vi "ProdaNG.TestValue.Set.vi"(8 "error in (no error)":errorcluster, 10 "TestValue":T1 {"minimum" format="%#.3f"; "maximum" format="%#.3f"}, 11 "dbHandleIn":i32) -> (0 "error out":errorcluster, 2 "TestValue out":T1 {"minimum" format="%#.3f"; "maximum" format="%#.3f"}, 3 "dbHandle":i32)   [LabVIEW 2016]
doc: "This function returns a product structure for a product, which is identified by a part and a serial number.\nImportant information: The field 'individual' was taken over from the field 'allgemein' of the legacy data directly. Because of this most products have the value 0 further on and only a few the value 1. \nParameter:\nhandle is an Integer, which is returned by the function Login() at the creation of a new connection.\nwabcoPartId is the Id of the part.\nserialNumber is the serial number of the product for the part above.\nproduct is a pointer on a product structure, which is filled if the returncode is 0. The structure must be defined in the calling program.\n\nReturncodes:\n0 No error\n< 0 ORACLE Error code\n6 (ERROR_INVALID_HANDLE) in case of an invalid handle\n1403 Record does not exist"
uses:
  Controls/ProdaNG.TestValue.ctl
  Controls/ProdaNG.TestValueSize.ctl
  prodllNG.dll
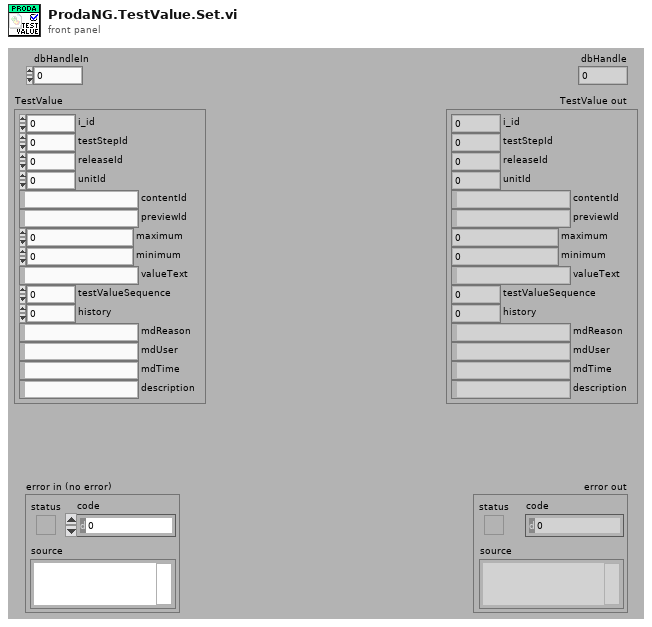
[diagram p1: front panel]
types:
  T1 = typedef "ProdaNG.TestValue.ctl" = cluster{"i_id":i32, "testStepId":i32, "releaseId":i32, "unitId":i32, "contentId":string, "previewId":string, "maximum":dbl, "minimum":dbl, "valueText":string, "testValueSequence":i32, "history":i32, "mdReason":string, "mdUser":string, "mdTime":string, "description":string}
  T2 = typedef "ProdaNG.TestValueSize.ctl" = cluster{"i_id":i32, "testStepId":i32, "releaseId":i32, "unitId":i32, "contentId":i32, "previewId":i32, "maximum":i32, "minimum":i32, "valueText":i32, "testValueSequence":i32, "history":i32, "mdReason":i32, "mdUser":i32, "mdTime":i32, "description":i32}
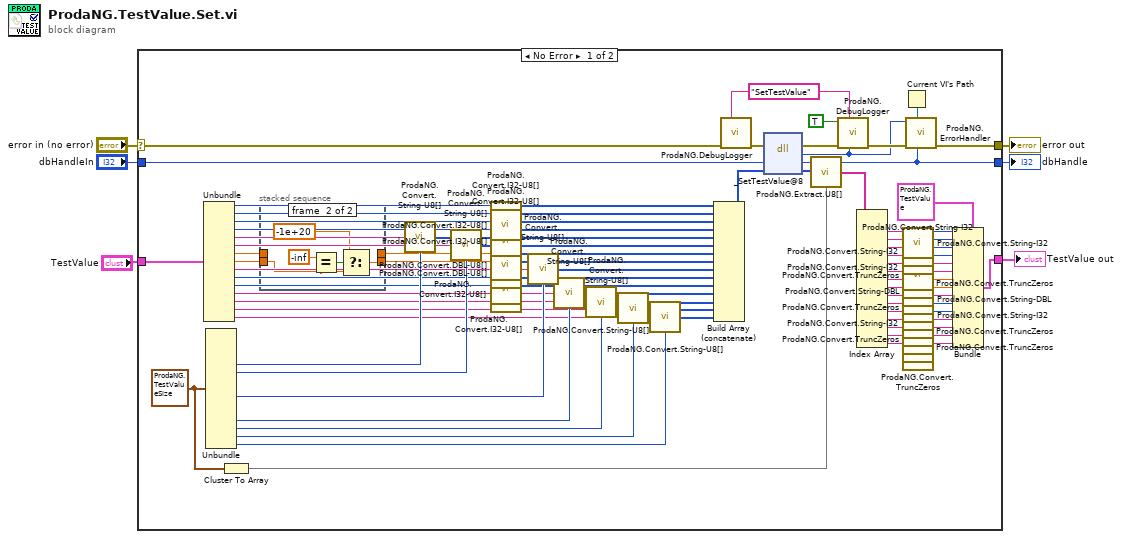
[diagram p0: block diagram]
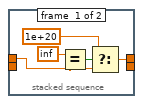
[diagram p2: hidden frame]
diagram:
  n1 = case shown="No Error" "error in (no error)" {
    selector: "error in (no error)" -> [w89 w106]
    tunnel: [w94 w106] -> w5
    tunnel: "dbHandleIn" -> [w91 w105]
    tunnel: [w92 w105] -> w3
    tunnel: "TestValue" -> [w58 _]
    tunnel: [w46 _] -> w2
    frame No Error {
      w31 = T2 {"i_id"=4, "testStepId"=4, "releaseId"=4, "unitId"=4, "contentId"=16, "previewId"=16, "maximum"=8, "minimum"=8, "valueText"=258, "testValueSequence"=4, "history"=4, "mdReason"=514, "mdUser"=22, "mdTime"=24, "description"=514} ("TestStepValueSize")
      w85 = "SetTestValue" ("cmd")
      n2 = Unbundle(w58) -> ("i_id"=w81:i32, "testStepId"=w82:i32, "releaseId"=w54:i32, "unitId"=w53:i32, "contentId"=w79:string, "previewId"=w50:string, "maximum"=w10:dbl, "minimum"=w9:dbl, "valueText"=w29:string, "testValueSequence"=w26:i32, "history"=w25:i32, "mdReason"=w22:string, "mdUser"=w20:string, "mdTime"=w16:string, "description"=w15:string)
      n3 = Unbundle(w31) -> ("contentId"=w76:i32, "previewId"=w49:i32, "valueText"=w27:i32, "mdReason"=w21:i32, "mdUser"=w17:i32, "mdTime"=w13:i32, "description"=w14:i32)  [unwired: 8 out]
      n4 = Cluster To Array(cluster=w31) -> (array=w55:i32[])
      n5 = stacked-sequence {
        tunnel: w10 -> [w95 _]
        tunnel: w9 -> [_ w100]
        tunnel: [w97 _] -> w8
        tunnel: [_ w101] -> w7
        frame #0 {
          n6 = Equal?(x=inf, y=w95) -> (x = y?=w96:bool)
          n7 = Select(t=1e+20, s=w96, f=w95) -> (s? t:f=w97:dbl)
        }
        frame #1 {
          n8 = Equal?(x=-inf, y=w100) -> (x = y?=w102:bool)
          n9 = Select(t=-1e+20, s=w102, f=w100) -> (s? t:f=w101:dbl)
        }
      }
      n10 = call "ProdaNG.Convert.String-U8[].vi"("Input String"=w79, "Size"=w76) -> ("Output"=w78:u8[])
      n11 = call "ProdaNG.Convert.String-U8[].vi"("Input String"=w50, "Size"=w49) -> ("Output"=w47:u8[])
      n12 = call "ProdaNG.Convert.I32-U8[].vi"("32bit integer"=w81) -> ("unsigned byte array"=w80:u8[])  [unwired: 10 in]
      n13 = call "ProdaNG.Convert.I32-U8[].vi"("32bit integer"=w82) -> ("unsigned byte array"=w83:u8[])  [unwired: 10 in]
      n14 = call "ProdaNG.Convert.I32-U8[].vi"("32bit integer"=w54) -> ("unsigned byte array"=w51:u8[])  [unwired: 10 in]
      n15 = call "ProdaNG.Convert.I32-U8[].vi"("32bit integer"=w53) -> ("unsigned byte array"=w52:u8[])  [unwired: 10 in]
      n16 = call "ProdaNG.Convert.DBL-U8[].vi"("dbl"=w8) -> ("unsigned byte array"=w77:u8[])  [unwired: 10 in]
      n17 = call "ProdaNG.Convert.DBL-U8[].vi"("dbl"=w7) -> ("unsigned byte array"=w30:u8[])  [unwired: 10 in]
      n18 = call "ProdaNG.Convert.I32-U8[].vi"("32bit integer"=w26) -> ("unsigned byte array"=w24:u8[])  [unwired: 10 in]
      n19 = call "ProdaNG.Convert.I32-U8[].vi"("32bit integer"=w25) -> ("unsigned byte array"=w23:u8[])  [unwired: 10 in]
      n20 = call "ProdaNG.Convert.String-U8[].vi"("Input String"=w29, "Size"=w27) -> ("Output"=w28:u8[])
      n21 = call "ProdaNG.Convert.String-U8[].vi"("Input String"=w22, "Size"=w21) -> ("Output"=w18:u8[])
      n22 = call "ProdaNG.Convert.String-U8[].vi"("Input String"=w20, "Size"=w17) -> ("Output"=w19:u8[])
      n23 = call "ProdaNG.Convert.String-U8[].vi"("Input String"=w16, "Size"=w13) -> ("Output"=w12:u8[])
      n24 = call "ProdaNG.Convert.String-U8[].vi"("Input String"=w15, "Size"=w14) -> ("Output"=w11:u8[])
      n25 = Build Array (concatenate)(w80, w83, w51, w52, w78, w47, w77, w30, w28, w24, w23, w18, w19, w12, w11) -> (w57:u8[])
      n26 = call "ProdaNG.DebugLogger.vi"("cmd"=w85, "error in (no error)"=w89) -> ("error out"=w88:errorcluster)  [unwired: 9 in]
      n27 = dll-call lib="D:/svn/LineTraceSystem/SOFTWARE/sources/Database/ProdaNG/prodllNG.dll" fn="_SetTestValue@8" ("ProDLL wrapper.dll:ProDLL_wrapper_GetWabcoParts_GetData")(error in=w88, "dbHandle"=w91, "testValuePtr"=w57) -> (error out=w87:errorcluster, "return type"=w84:i32, "dbHandle"=w92:i32, "testValuePtr"=w56:u8[])  [unwired: 2 in, 1 out]
      n28 = call "ProdaNG.Extract.U8[].vi"("unsigned byte array"=w56, "Sizes"=w55) -> ("Elements"=w75:string[])
      n29 = call "ProdaNG.DebugLogger.vi"("return type"=w84, "cmd"=w85, "error in (no error)"=w87, "done? (F)"=TRUE) -> ("error out"=w86:errorcluster)  [unwired: 7 in]
      n30 = Index Array(array=w75) -> (element #1=w74:string, element #2=w71:string, element #3=w70:string, element #4=w64:string, element #5=w61:string, element #6=w60:string, element #7=w65:string, element #8=w67:string, element #9=w44:string, element #10=w43:string, element #11=w42:string, element #12=w39:string, element #13=w37:string, element #14=w35:string, element #15=w34:string)  [unwired: 15 in]
      n31 = Current VI's Path() -> (path=w93:path)
      n32 = call "ProdaNG.Convert.String-I32.vi"("unsigned byte string"=w74) -> ("32bit integer"=w73:i32)  [unwired: 10 in]
      n33 = call "ProdaNG.Convert.String-I32.vi"("unsigned byte string"=w71) -> ("32bit integer"=w72:i32)  [unwired: 10 in]
      n34 = call "ProdaNG.Convert.String-I32.vi"("unsigned byte string"=w70) -> ("32bit integer"=w69:i32)  [unwired: 10 in]
      n35 = call "ProdaNG.Convert.String-I32.vi"("unsigned byte string"=w64) -> ("32bit integer"=w63:i32)  [unwired: 10 in]
      n36 = call "ProdaNG.Convert.TruncZeros.vi"("string with \\0s"=w61) -> ("LV string"=w62:string)  [unwired: 10 in]
      n37 = call "ProdaNG.Convert.TruncZeros.vi"("string with \\0s"=w60) -> ("LV string"=w59:string)  [unwired: 10 in]
      n38 = call "ProdaNG.Convert.String-DBL.vi"("unsigned byte string"=w65) -> ("dbl integer"=w66:dbl)  [unwired: 10 in]
      n39 = call "ProdaNG.Convert.String-DBL.vi"("unsigned byte string"=w67) -> ("dbl integer"=w68:dbl)  [unwired: 10 in]
      n40 = call "ProdaNG.Convert.TruncZeros.vi"("string with \\0s"=w44) -> ("LV string"=w45:string)  [unwired: 10 in]
      n41 = call "ProdaNG.Convert.String-I32.vi"("unsigned byte string"=w43) -> ("32bit integer"=w41:i32)  [unwired: 10 in]
      n42 = call "ProdaNG.Convert.String-I32.vi"("unsigned byte string"=w42) -> ("32bit integer"=w40:i32)  [unwired: 10 in]
      n43 = call "ProdaNG.Convert.TruncZeros.vi"("string with \\0s"=w39) -> ("LV string"=w38:string)  [unwired: 10 in]
      n44 = call "ProdaNG.Convert.TruncZeros.vi"("string with \\0s"=w37) -> ("LV string"=w36:string)  [unwired: 10 in]
      n45 = call "ProdaNG.Convert.TruncZeros.vi"("string with \\0s"=w35) -> ("LV string"=w33:string)  [unwired: 10 in]
      n46 = call "ProdaNG.Convert.TruncZeros.vi"("string with \\0s"=w34) -> ("LV string"=w32:string)  [unwired: 10 in]
      n47 = call "ProdaNG.ErrorHandler.vi"("dbHandleIn"=w92, "Path"=w93, "error in"=w86, "output_parameter"=w84) -> ("error out"=w94:errorcluster)  [unwired: 7 in]
      n48 = Bundle(cluster=T1 {"i_id"=0, "testStepId"=0, "releaseId"=0, "unitId"=0, "contentId"="", "previewId"="", "maximum"=0.0, "minimum"=0.0, "valueText"="", "testValueSequence"=0, "history"=0, "mdReason"="", "mdUser"="", "mdTime"="", "description"=""} ("TestStepValue"), "i_id"=w73, "testStepId"=w72, "releaseId"=w69, "unitId"=w63, "contentId"=w62, "previewId"=w59, "maximum"=w66, "minimum"=w68, "valueText"=w45, "testValueSequence"=w41, "history"=w40, "mdReason"=w38, "mdUser"=w36, "mdTime"=w33, "description"=w32) -> (w46:T1)
    }
    frame Error {
    }
  }
  "error out" <- w5
  "dbHandle" <- w3
  "TestValue out" <- w2
